vi "TCP_WriteRead.vi"(8 "error in":errorcluster, 9 "bytes to read":i32=10, 10 "Parameter 1":string="VE", 11 "connection ID":refnum<k5>) -> (0 "error out":errorcluster, 2 "DataOut":string, 3 "TCP Network Connection out":refnum<k5>)   [LabVIEW 2019]
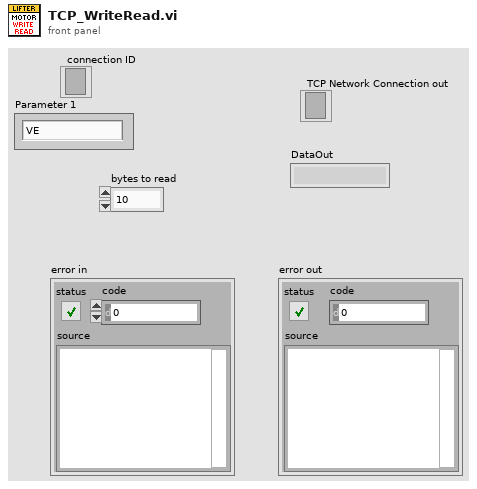
[diagram p1: front panel]
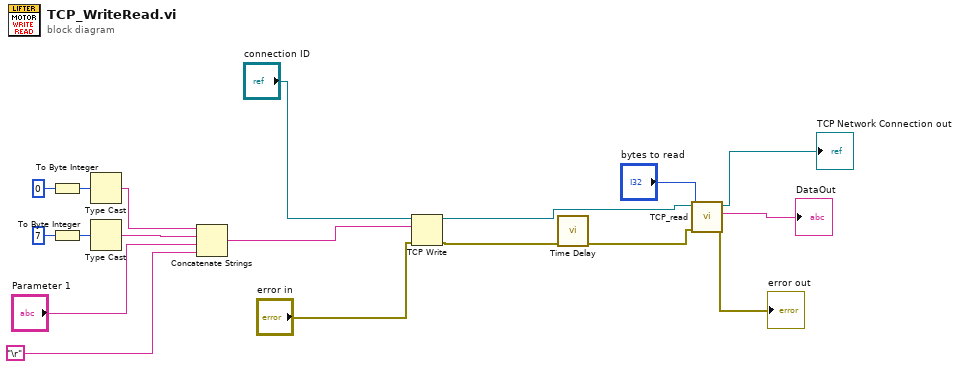
[diagram p0: block diagram]
diagram:
  n1 = To Byte Integer(number=i8 0) -> (8bit integer=w10:i8)
  n2 = To Byte Integer(number=i8 7) -> (8bit integer=w13:i8)
  n3 = Type Cast(x=w10) -> (*(type *) &x=w11:string)  [unwired: 1 in]
  n4 = Type Cast(x=w13) -> (*(type *) &x=w12:string)  [unwired: 1 in]
  n5 = Concatenate Strings(w11, w12, "Parameter 1", "\r") -> (w7:string)
  n6 = TCP Write(connection ID="connection ID", data in=w7, error in (no error)="error in") -> (connection ID out=w3:refnum<k5>, error out=w4:errorcluster)  [unwired: 1 in, 1 out]
  n7 = call "Time Delay"("error in (no error)"=w4) -> ("error out"=w15:errorcluster)  [unwired: 10 in]
  n8 = call "TCP_read.vi"("error in (no error)"=w15, "bytes to read"="bytes to read", "TCP Network Connection in"=w3) -> ("error out"=→"error out":errorcluster, "DataOut"=→"DataOut":string, "TCP Network Connection out"=→"TCP Network Connection out":refnum<k5>)  [unwired: 6 in]
